vi "iteration.vi"(0 "GUI refnum cluster":T30, 1 "all settings":T1={"Variable Settings"={"Measurements per Iteration"=0, "Local Data Path"=path "", "Experiment description suffix for filename (no spaces please)"="", "Network Data Path"=path "", "Copy data to network"=FALSE, "Measurement Timeout (ms)"=0, "Independent Variables"=[], "Dependent Variables"=[], "Run Test Mode"=FALSE}, "HSDIO Settings"={"Enable HSDIO Pulses"=FALSE, "Resource Name"="", "Clock Rate"=0.0, "units/sec (ms=1000)"=0.0, "Array of Script Triggers"=[], "Channels Control"=[], "Pulse Generation Script"="", "Directory to look for waveform files"=path "", "Start Trigger"={"Wait for start trigger?"=FALSE, "source (PFI 0)"="", "edge (rising)"=0}, "Hardware alignment quantum\n(in samples)"=0, "Use file script"=FALSE, "Base path for script"=path "", "filename for script"=""}, "DAQmx Pulse Settings"={"Enable DAQmx Pulses"=FALSE, "DAQmx Physical Channels"="", "Clock Rate"=0.0, "units/sec (ms=1000)"=0.0, "Start Trigger"={"Wait for start trigger?"=FALSE, "source"="", "edge"=0}, "Timing Sequence Control"=[]}, "DDS Settings"={"Enable DDS"=FALSE, "Array of DDS Boxes"=[]}, "Camera settings"={"Analog Gain (0-5)"=0, "Frame Grabber acquisition region\n(left, top, right, bottom)"=[], "Exposure Time"=0.0, "EM Gain (0-255)"=0, "Trigger Polarity"="", "External Trigger Mode"="", "Scan Speed"="", "External Trigger Source"="", "Scan Mode"="", "Super Pixel Binning\n(if enabled in Scan Mode)"="", "Camera Sub-array acquisition region\n(if enabled in scan mode)"={"Left"=0, "Top"=0, "Width"=0, "Height"=0}, "Use camera?"=FALSE, "# image buffers"=0, "Regions of Interest (Left, Top, Right, Bottom)"=[], "Background Regions (Left, Top, Right, Bottom)"=[], "shots per measurement"=0, "Photoelectron Scaling"=0.0, "Force images to U16"=FALSE}, "Counter Settings"={"Enable Counters"=FALSE, "Array of Counter Settings"=[]}, "Filter Cluster"={"Counter Filter thresholds"=[], "Data Filters\nROI Minimum Thresholds"=[]}, "Analog Output Parameters"={"Enable Analog Out?"=TRUE, "Physical Channel"="PXI1Slot2/ao0:2", "Minimum Value"=-10.0, "Maximum Value"=10.0, "Samples per second"="", "Total AO Time (seconds)"="p", "Analog Output Equations for each Channel"=[], "Start Trigger"={"Wait for start trigger?"=FALSE, "source"="/Dev1/PFI0", "edge"=10280}}, "Notes"="", "HP83623A Generator Settings Array"=[], "Iteration Graph Settings"={"Plot Regions"="", "Plot Shots"=""}, "PI Piezo Settings"={"Enable"=FALSE, "Array of Piezo Controllers"=[]}, "Andor settings"={"Andor Path"=path "", "Copy any Andor files"=FALSE, "Wait time before copying Andor files (ms)"=0}, "Measurement Chart Settings"={"Which regions to plot (comma separated)"="", "Which shot to plot"=0}, "HP8662A Synthesized Signal Generator Array"=[], "HP83712B Synthesized CW Generator Array"=[], "TTL input"={"Enable"=FALSE, "lines"=""}} {"Variable Settings"."Independent Variables"."# steps" min=1 step=1; "Variable Settings"."Measurements per Iteration" min=1 step=1; "HSDIO Settings"."Hardware alignment quantum\n(in samples)" min=1 step=1; "HSDIO Settings"."Array of Script Triggers"."level" items=["High Level"=34, "Low Level"=35]; "HSDIO Settings"."Array of Script Triggers"."edge" items=["Rising Edge"=12, "Falling Edge"=13]; "HSDIO Settings"."Start Trigger"."edge (rising)" items=["Rising Edge"=12, "Falling Edge"=13]; "HSDIO Settings"."Clock Rate" min=0.0 max=200000000.0 format="%.2p"; "DAQmx Pulse Settings"."Start Trigger"."edge" items=["Rising"=10280, "Falling"=10171]; "DAQmx Pulse Settings"."Clock Rate" min=0.0 max=200000000.0 format="%.2p"; "Camera settings"."shots per measurement" min=0 step=1; "Camera settings"."Background Regions (Left, Top, Right, Bottom)" min=0 max=512 step=1; "Camera settings"."Regions of Interest (Left, Top, Right, Bottom)" min=0 max=512 step=1; "Camera settings"."# image buffers" min=0 step=1; "Camera settings"."Camera Sub-array acquisition region\n(if enabled in scan mode)"."Height" min=16 max=512 step=16; "Camera settings"."Camera Sub-array acquisition region\n(if enabled in scan mode)"."Width" min=16 max=512 step=16; "Camera settings"."Camera Sub-array acquisition region\n(if enabled in scan mode)"."Top" max=496 step=16; "Camera settings"."Camera Sub-array acquisition region\n(if enabled in scan mode)"."Left" max=496 step=16; "Camera settings"."Frame Grabber acquisition region\n(left, top, right, bottom)" min=0 max=512 step=1; "Camera settings"."Analog Gain (0-5)" max=5 step=1; "Counter Settings"."Array of Counter Settings"."Binwidth (ms)" format="%0.2f"; "Analog Output Parameters"."Start Trigger"."edge" items=["Rising"=10280, "Falling"=10171]; "Analog Output Parameters"."Maximum Value" format="%0.2f"; "Analog Output Parameters"."Minimum Value" format="%0.2f"}, 2 "Variable Settings Refnum":refnum<vi>, 7 "error in (no error)":errorcluster, 8 "Image Display Refnum Array":refnum<vi>[](array[refnum]), 12 "Camera Temperature Refnum":refnum<vi>, 14 "HSDIO Status Refnum":refnum<vi>, 16 "# intervals (mutli-shot)":i32=128, 17 "Notes Refnum":refnum<vi>, 22 "Hamamatsu_C9100-13.lvclass":refnum<class "Hamamatsu_C9100-13.lvclass">, 26 "Variable Status Refnum":refnum<vi>) -> (20 "Array of ROI sums":dbl[][][][](array[numeric])=[[[[-878.86977886979]]]], 21 "Image Array for whole experiment":T35[][][](array[plugin-control]) caption="(Cycles, Iterations, Measurements, Shots, scaling above)", 23 "Histogram of ROI Sum over All Images for last ROI":T33, 24 "Average of All Images from experiment":T35(plugin-control) caption="Average of All Images (dynamically scaled)", 25 "Camera out":refnum<class "Hamamatsu_C9100-13.lvclass">, 27 "error out":errorcluster)   [LabVIEW 2012]
doc: "I Description:\nThis example uses a script to manage the generation of a dynamic pattern at a specified clock rate.\n\nII Instructions for Running:\n1. Enter the digital channels on the hardware device to generate digital pattern in the Channel List control.\n2. Specify the clock rate for the generation in the Clock Rate control.\n3. Click the Stop button when you want to stop the generation\n\nIII Block Diagram Steps:\n1. Initialize for a generation session.\n2. Assign specified channels in Channel List for dynamic operation.\n3. Configure the Sample clock to use the onboard clock, and configure the clock rate.\n4. Set the generation mode to Scripted.\n5. Query the Data Width property to determine which Write function to use.\nNote: Different devices have different default values for the Data Width property. If you know the Data Width of your device, you may omit the property node and case structure.\n6. Write digital patterns to the onboard memory of the digital device.\n7. Write the script to the onboard memory.\n8. Initiate dynamic pattern generation.\n9. Wait until the Stop button is clicked or an error occurs, and exit the While loop. \n The niHSDIO Is Done VI is used in the while loop to check only for errors.\n10. Abort generation and close the session.\n\nIV I/O Connections Overview:\nMake connections from output terminals to match the channels specified by Channel List. In this example, the digital pattern is generated from the first 16 digital channels of the device."
uses:
  ExperimentVariables/ExperimentVariables.lvclass
  DAQmx_pulse_out/DAQmx_pulse_out.lvclass
  HSDIO/HSDIO.lvclass
  Analog_output/Analog_Output.lvclass
  Camera/Hamamatsu_C9100-13/Hamamatsu_C9100-13.lvclass
  Counter/Counter.lvclass
  GPIB/GPIB.lvclass
  Analog_output/AO_settings.ctl
  Camera/Hamamatsu_C9100-13/camera_setup.ctl
  DDS drivers v3/DDS RAM mode.ctl
  <vilib>/ni845x/ni845x.llb/ni845xControl.ctl
  <instrlib>/niHSDIO/niHSDIO.llb/niHSDIO_ctl Trigger Script - trigID Values (Ring).ctl
  <instrlib>/niHSDIO/niHSDIO.llb/niHSDIO_ctl Trigger DigEdge - Edge Values (Ring).ctl
  <instrlib>/niHSDIO/niHSDIO.llb/niHSDIO_ctl Trigger Source Values (Ring).ctl
  ExperimentVariables/Variable_Settings.ctl
  Counter/Counter_Settings_Control.ctl
  HSDIO/HSDIO_settings.ctl
  DAQmx_pulse_out/settings.ctl
  <instrlib>/niHSDIO/niHSDIO.llb/niHSDIO_ctl Trigger DigLvl - Level Values (Ring).ctl
  histogram.ctl
  gui_refnum.ctl
  Counter/counter_graph_refnums.ctl
  filters/filters.ctl
  gui_execution_controls.ctl
  DDS drivers v3/Array_of_DDS_Boxes.ctl
  DDS drivers v3/DDS_box_device_reference.ctl
  DDS drivers v3/DDS_box_cluster.ctl
  DDS/DDS_Settings_Cluster.ctl
  config_file_io/all_settings.ctl
  ExperimentVariables/Variable_Status.ctl
  GPIB/HP83623A_RF_Generator/HP83623A_settings.ctl
  GPIB/HP83623A_RF_Generator/HP83623A_RF_Generator.lvclass
  PI_piezo/settings.ctl
  PI_piezo/status.ctl
  Camera/Andor/Andor_settings.ctl
  gui/measurement_graph.ctl
  GPIB/RF_Generator_settings.ctl
  GPIB/RF_Generator_settings_array.ctl
  DDS drivers v3/DDS_profile.ctl
  DDS drivers v3/DDS_channel.ctl
  DDS/DDS.lvclass
  DDS drivers v3/array_of_DDS_profiles.ctl
  DDS drivers v3/array_of_DDS_channels.ctl
  ExperimentVariables/current_variables_table.ctl
  TTL_input/TTL_input_settings.ctl
  TTL_input/TTL_input.lvclass
panel:
  out "Counter out":refnum<class "Counter.lvclass">
  out "HSDIO":refnum<class "HSDIO.lvclass">
  out "Run Test Mode":bool
  in  "Tab Control":T34(tab)=enum."Filters"
  # "Parameters will be evaluated once at the beginning of the experiment from top to bottom, \nso any parameter may depend on all those above it.\nVariables will be evaluated each iteration.\nParameters and Variables may be used in various other experiment settings, as noted.\nSee LabView Help -> Formula Node and Expression Node Functions for a list of available functions."
  # "Parameters will be evaluated once at the beginning of the experiment from top to bottom, \nso any parameter may depend on all those above it.\nVariables will be evaluated each iteration.\nParameters and Variables may be used in various other experiment settings, as noted.\nSee LabView Help -> Formula Node and Expression Node Functions for a list of available functions."
  # "Regions of Interest -->"
  # "Shots\n   |\n  V"
  # "Counters -->"
  # "Counter\n    bins\n       |\n      V"
  # "You may use formulas here.  If 't' is not specified in the variable or parameter tables, it will be used here as time in seconds.\nIn addition to the usual functions (sin(), cos(), etc.) you may also use spike(), square() and step(), \nNote, analog output will continue until Total AO Time runs out, or Measurement Timeout is reached, \neven if HSDIO pulses or DAQmx pulses have finished."
  # "Notes will be auto-evaluated and will be saved with comments in each experiment directory."
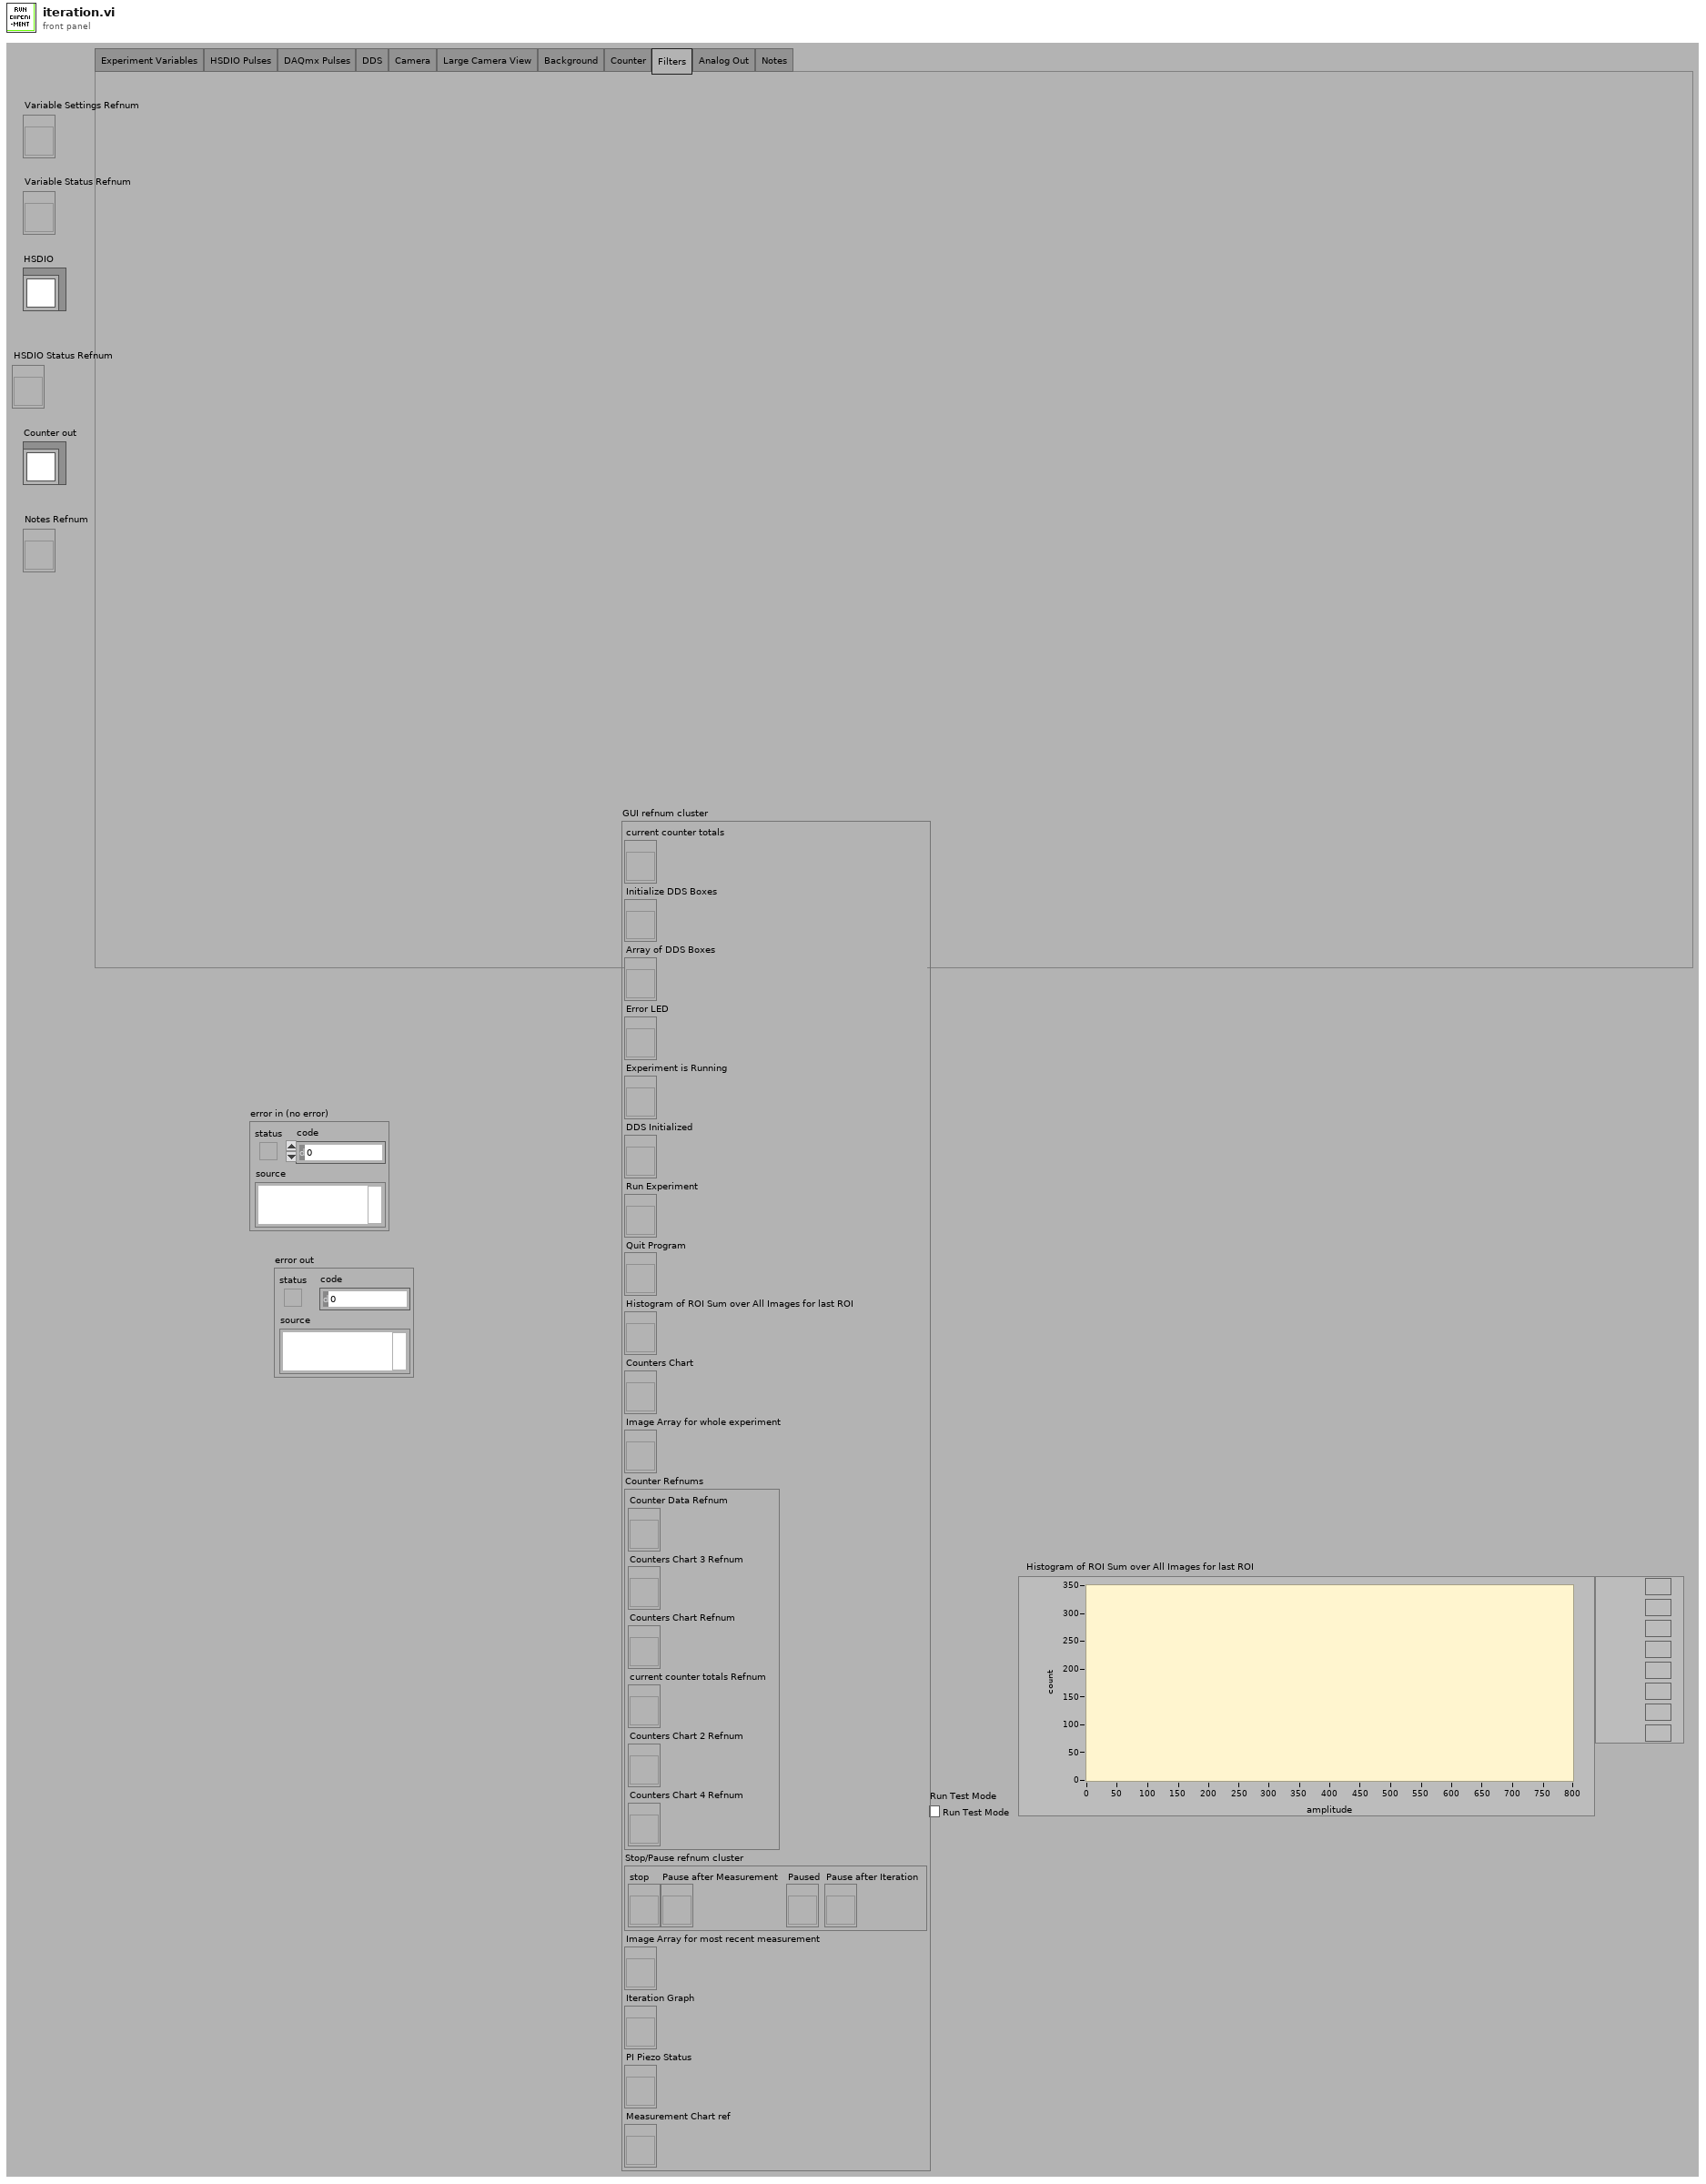
[diagram p1: front panel]
types:
  T1 = typedef "all_settings.ctl" = cluster{"Variable Settings":T2, "HSDIO Settings":T3, "DAQmx Pulse Settings":T8, "DDS Settings":T9, "Camera settings":T19, "Counter Settings":T20, "Filter Cluster":T21, "Analog Output Parameters":T22, "Notes":string, "HP83623A Generator Settings Array":T23, "Iteration Graph Settings":cluster{"Plot Regions":string, "Plot Shots":string}, "PI Piezo Settings":T24, "Andor settings":T25, "Measurement Chart Settings":T26, "HP8662A Synthesized Signal Generator Array":T27, "HP83712B Synthesized CW Generator Array":T27, "TTL input":T29}
  T2 = typedef "ExperimentVariables.lvclass/Variable_Settings.ctl" = cluster{"Measurements per Iteration":i32, "Local Data Path":path, "Experiment description suffix for filename (no spaces please)":string, "Network Data Path":path, "Copy data to network":bool, "Measurement Timeout (ms)":u32, "Independent Variables":cluster{"Description":string, "Name (a,a0...a9)":string, "min":dbl, "max":dbl, "# steps":u32}[], "Dependent Variables":cluster{"Description":string, "Name (a,a0...a9)":string, "Equation":string, "Result":dbl}[], "Run Test Mode":bool}
  T3 = typedef "HSDIO.lvclass/HSDIO_settings.ctl" = cluster{"Enable HSDIO Pulses":bool, "Resource Name":refnum<k15>, "Clock Rate":dbl, "units/sec (ms=1000)":dbl, "Array of Script Triggers":cluster{"trigger id (script trigger 0)":T4, "source (PFI 0)":T5, "Trigger Type":enum32{"Edge", "Level"}, "edge":T6, "level":T7}[], "Channels Control":string[][], "Pulse Generation Script":string, "Directory to look for waveform files":path, "Start Trigger":cluster{"Wait for start trigger?":bool, "source (PFI 0)":T5, "edge (rising)":T6}, "Hardware alignment quantum\n(in samples)":u16, "Use file script":bool, "Base path for script":path, "filename for script":string}
  T4 = typedef "niHSDIO_ctl Trigger Script - trigID Values (Ring).ctl" = string
  T5 = typedef "niHSDIO_ctl Trigger Source Values (Ring).ctl" = string
  T6 = typedef "niHSDIO_ctl Trigger DigEdge - Edge Values (Ring).ctl" = i32
  T7 = typedef "niHSDIO_ctl Trigger DigLvl - Level Values (Ring).ctl" = i32
  T8 = typedef "DAQmx_pulse_out.lvclass/settings.ctl" = cluster{"Enable DAQmx Pulses":bool, "DAQmx Physical Channels":tag, "Clock Rate":dbl, "units/sec (ms=1000)":dbl, "Start Trigger":cluster{"Wait for start trigger?":bool, "source":tag, "edge":i32}, "Timing Sequence Control":string[][]}
  T9 = typedef "DDS_Settings_Cluster.ctl" = cluster{"Enable DDS":bool, "Array of DDS Boxes":T10}
  T10 = typedef "Array_of_DDS_Boxes.ctl" = T11[]
  T11 = typedef "DDS_box_cluster.ctl" = cluster{"DDS box device reference":T12, "Array of DDS Channels (4)":T14, "Enable":bool, "Description":string}
  T12 = typedef "DDS_box_device_reference.ctl" = cluster{"NI USB-8451 device reference":T13, "DIO port":u8, "Serial Clock Rate [kHz]":u16}
  T13 = typedef "ni845xControl.ctl" = refnum<k21>
  T14 = typedef "DDS.lvclass/array_of_DDS_channels.ctl" = T15[]
  T15 = typedef "DDS.lvclass/DDS_channel.ctl" = cluster{"Power":bool, "Channel Parameters":cluster{"Ref Clock Rate [kHz]":dbl, "Full Scale Output\nPower [dBm]":dbl}, "RAM Enable":bool, "RAM Dest Type":u8, "RAM Default":cluster{"Frequency [MHz]":string, "Amplitude [dBm]":string, "Phase Offset [rad]":string}, "Array of DDS Profiles (8)":T16, "Description":string}
  T16 = typedef "DDS.lvclass/array_of_DDS_profiles.ctl" = T17[]
  T17 = typedef "DDS_profile.ctl" = cluster{"Single Tone":cluster{"Frequency [MHz]":string, "Amplitude [dBm]":string, "Phase Offset [rad]":string}, "RAM Mode ":T18, "Zero-crossing":bool, "No Dwell High":bool, "Function/Static":bool, "RAM Function Settings":string[], "RAM Static Array":dbl[], "Description":string}
  T18 = typedef "DDS RAM mode.ctl" = enum16{"Direct Switch", "Ramp Up", "Bidirectional Ramp", "Continuous Bidirectional Ramp", "Continuous Recirculate", "Direct Switch 2", "Direct Switch 3", "Direct Switch 4"}
  T19 = typedef "Hamamatsu_C9100-13.lvclass/camera_setup.ctl" = cluster{"Analog Gain (0-5)":u8, "Frame Grabber acquisition region\n(left, top, right, bottom)":i32[], "Exposure Time":dbl, "EM Gain (0-255)":u8, "Trigger Polarity":string, "External Trigger Mode":string, "Scan Speed":string, "External Trigger Source":string, "Scan Mode":string, "Super Pixel Binning\n(if enabled in Scan Mode)":string, "Camera Sub-array acquisition region\n(if enabled in scan mode)":cluster{"Left":u16, "Top":u16, "Width":u16, "Height":u16}, "Use camera?":bool, "# image buffers":i32, "Regions of Interest (Left, Top, Right, Bottom)":i32[][], "Background Regions (Left, Top, Right, Bottom)":i32[][], "shots per measurement":i32, "Photoelectron Scaling":dbl, "Force images to U16":bool}
  T20 = typedef "Counter.lvclass/Counter_Settings_Control.ctl" = cluster{"Enable Counters":bool, "Array of Counter Settings":cluster{"Counter Channel":tag, "Time-Bin Clock Channel":tag, "Binwidth (ms)":dbl}[]}
  T21 = typedef "filters.ctl" = cluster{"Counter Filter thresholds":u32[][], "Data Filters\nROI Minimum Thresholds":u64[][]}
  T22 = typedef "Analog_Output.lvclass/AO_settings.ctl" = cluster{"Enable Analog Out?":bool, "Physical Channel":tag, "Minimum Value":dbl, "Maximum Value":dbl, "Samples per second":string, "Total AO Time (seconds)":string, "Analog Output Equations for each Channel":string[], "Start Trigger":cluster{"Wait for start trigger?":bool, "source":tag, "edge":i32}}
  T23 = typedef "HP83623A_RF_Generator.lvclass/HP83623A_settings.ctl" = cluster{"Frequency (Hz)":string, "Power (dBm)":string, "Enabled":bool, "initialized":bool, "RF Output On/Off":bool, "External Trigger?":bool, "VISA Session":refnum<visa-resource-name>, "Generator Name":string}[]
  T24 = typedef "settings.ctl" = cluster{"Enable":bool, "Array of Piezo Controllers":cluster{"Enable":bool, "Serial No.":string, "Array of Piezo Channels":cluster{"Servo":bool, "Set Position":string}[]}[]}
  T25 = typedef "Andor_settings.ctl" = cluster{"Andor Path":path, "Copy any Andor files":bool, "Wait time before copying Andor files (ms)":u16}
  T26 = typedef "measurement_graph.ctl" = cluster{"Which regions to plot (comma separated)":string, "Which shot to plot":u8}
  T27 = typedef "GPIB.lvclass/RF_Generator_settings_array.ctl" = T28[]
  T28 = typedef "GPIB.lvclass/RF_Generator_settings.ctl" = cluster{"Enable":bool, "Description":string, "GPIB channel #":u8, "Frequency (MHz)":string, "Power (dBm)":string}
  T29 = typedef "TTL_input.lvclass/TTL_input_settings.ctl" = cluster{"Enable":bool, "lines":tag}
  T30 = typedef "gui_refnum.ctl" = cluster{"current counter totals":refnum<vi>, "Initialize DDS Boxes":refnum<vi>, "Array of DDS Boxes":refnum<vi>, "Error LED":refnum<vi>, "Experiment is Running":refnum<vi>, "DDS Initialized":refnum<vi>, "Run Experiment":refnum<vi>, "Quit Program":refnum<vi>, "Histogram of ROI Sum over All Images for last ROI":refnum<vi>, "Counters Chart":refnum<vi>, "Image Array for whole experiment":refnum<vi>, "Counter Refnums":T31, "Stop/Pause refnum cluster":T32, "Image Array for most recent measurement":refnum<vi>, "Iteration Graph":refnum<vi>, "PI Piezo Status":refnum<vi>, "Measurement Chart ref":refnum<vi>}
  T31 = typedef "counter_graph_refnums.ctl" = cluster{"Counter Data Refnum":refnum<vi>, "Counters Chart 3 Refnum":refnum<vi>, "Counters Chart Refnum":refnum<vi>, "current counter totals Refnum":refnum<vi>, "Counters Chart 2 Refnum":refnum<vi>, "Counters Chart 4 Refnum":refnum<vi>}
  T32 = typedef "gui_execution_controls.ctl" = cluster{"stop":refnum<vi>, "Pause after Measurement":refnum<vi>, "Paused":refnum<vi>, "Pause after Iteration":refnum<vi>}
  T33 = typedef "histogram.ctl" = cluster{"X Values":dbl[], "Histogram: h(x)":i32[]}[]
  T34 = enum32{"Experiment Variables", "HSDIO Pulses", "DAQmx Pulses", "DDS", "Camera", "Large Camera View", "Background", "Counter", "Filters", "Analog Out", "Notes"}
  T35 = typedef "IMAQ Image.ctl" = refnum<image>
  T36 = enum16{"reset", "experiment start", "experiment end", "quit"}
  T37 = cluster{"Plot Regions":string, "Plot Shots":string}
  T38 = cluster{"Global Rectangle":i32[], "Contours":cluster{"Contour Type":u32, "ROI Type":u32, "Points":i32[]}[]}
  T39 = cluster{"X Values":dbl[], "Histogram: h(x)":i32[]}[]
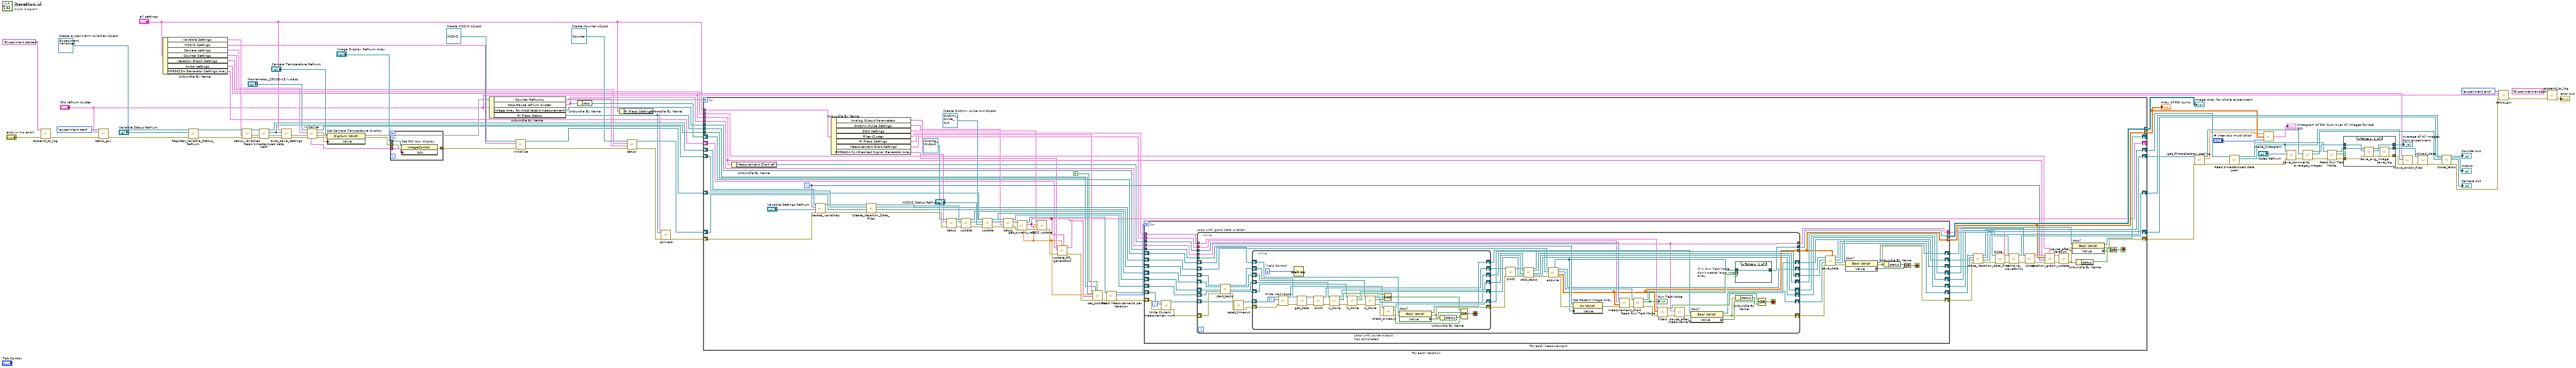
[diagram p0: block diagram]
diagram:
  w49 = refnum<class "Counter.lvclass"> refnum  # Create Counter object
  w77 = refnum<class "HSDIO.lvclass"> refnum  # Create HSDIO object
  w53 = refnum<class "ExperimentVariables.lvclass"> refnum  # Create experiment variables object
  n1 = call "append_to_log.vi"("error in"="error in (no error)", "string"="Experiment started") -> ("error out"=w58:errorcluster)  [unwired: 9 in]
  n2 = call "setup_gui.vi"("Enum"=T36."experiment start", "GUI refnum cluster"="GUI refnum cluster", "error in (no error)"=w58) -> ("error out"=w51:errorcluster)  [unwired: 12 in]
  n3 = Unbundle By Name("all settings") -> ("Variable Settings"=w18:T2, "HSDIO Settings"=w17:T3, "Camera settings"=w16:T19, "Counter Settings"=w15:T20, "Iteration Graph Settings"=w12:T37, "Andor settings"=w3:T25, "HP83623A Generator Settings Array"=w1:T23)
  n4 = call-dynamic "Register_Variable_Status_Refnum.vi"("error in (no error)"=w51, "Variable Status Refnum"="Variable Status Refnum", "ExperimentVariables in"=w53) -> ("error out"=w50:errorcluster, "ExperimentVariables out"=w52:refnum<class "ExperimentVariables.lvclass">)  [unwired: 7 in]
  n5 = call "setup_variables.vi"("error in (no error)"=w50, "Variable Settings"=w18, 11:w52) -> ("error out"=w39:errorcluster, 1:w79, "ExperimentVariables out"=w41:refnum<class "ExperimentVariables.lvclass">)  [unwired: 6 in]
  n6 = call-dynamic "Read timestamped data path.vi"("error in (no error)"=w39, "ExperimentVariables in"=w41) -> ("error out"=w19:errorcluster, "Specific Data Files Path"=w6:path, "ExperimentVariables out"=w40:refnum<class "ExperimentVariables.lvclass">)  [unwired: 7 in]
  n7 = call "auto_save_settings.vi"("error in"=w19, "base path"=w6, "all settings"="all settings") -> ("error out"=w14:errorcluster)  [unwired: 8 in]
  n8 = call-dynamic "initialize.vi"("error in (no error)"=w14, "Camera Setup"=w16, "Hamamatsu_C9100-13 in"="Hamamatsu_C9100-13.lvclass") -> ("error out"=w63:errorcluster, "Camera Temperature"=w64:dbl, "Hamamatsu_C9100-13 out"=w70:refnum<class "Hamamatsu_C9100-13.lvclass">, "ROI"=w71:T38)  [unwired: 5 in]
  n9 = property on="Set Camera Temperature Display" class="DigNum (strict)"(reference="Camera Temperature Refnum", error in=w63, "Value"=w64) -> (error out=w62:errorcluster)  [unwired: 1 out]
  n10 = for {
    tunnel: "Image Display Refnum Array" -> [w87] mode=indexing
    tunnel: w71 -> [w86]
    tunnel: w62 -> [w85]
    tunnel: [w84] -> w72
    n11 = property on="Set ROI box display" class="ImageControl"(reference=w87, error in=w85, "ROI"=w86) -> (error out=w84:errorcluster)  [unwired: 1 out]
  }
  n12 = Unbundle By Name("GUI refnum cluster") -> ("Counter Refnums"=w22:T31, "Stop/Pause refnum cluster"=w21:T32, "Image Array for most recent measurement"=w20:refnum<vi>, "PI Piezo Status"=w7:refnum<vi>)
  n13 = call "Initialize.vi"("error in (no error)"=w72, "HSDIO Settings"=w17, 11:w77) -> ("error out"=w48:errorcluster, "HSDIO out"=w76:refnum<class "HSDIO.lvclass">)  [unwired: 7 in]
  n14 = Unbundle By Name(w21) -> ("stop"=w61:refnum<vi>)
  n15 = Unbundle By Name("all settings") -> ("PI Piezo Settings"=w9:T24)
  n16 = call "setup.vi"("error in (no error)"=w48, "Counter Refnums"=w22, "Counter Settings"=w15, 11:w49) -> ("error out"=w11:errorcluster, "Counter out"=w47:refnum<class "Counter.lvclass">)  [unwired: 6 in]
  n17 = call "connect.vi"("PI Piezo Settings"=w9, "PI Piezo Status"=w7, "error in"=w11) -> ("error out"=w8:errorcluster)  [unwired: 16 in]
  n18 = for "For each Iteration" {
    N: w79 -> [_]
    shift-right: [w140] -> w27
    shift-left: w8 -> [w166]
    tunnel: [w108] -> w68 mode=indexing
    shift-right: [w162] -> w78
    shift-left: w76 -> [w165]
    shift-right: [w121] -> w80
    shift-left: w47 -> [w131]
    shift-right: [w124] -> w44
    shift-left: w40 -> [w167]
    tunnel: [w136] -> w75 mode=indexing
    shift-right: [w109] -> w28
    shift-left: w70 -> [w130]
    shift-right: [w138] -> _
    shift-left: w61 -> [w137]
    tunnel: w21 -> [w120]
    tunnel: w20 -> [w119]
    tunnel: "all settings" -> [w116]
    tunnel: "GUI refnum cluster" -> [w97]
    tunnel: w12 -> [w104]
    tunnel: w7 -> [w102]
    tunnel: w6 -> [w98]
    shift-right: [w89] -> _
    shift-left: w1 -> [w90]
    i -> [w105]
    stop <- w169 stop-if-true
    w160 = refnum<class "DAQmx_pulse_out.lvclass"> refnum  # Create DAQmx pulse out object
    n19 = Unbundle By Name(w97) -> ("Measurement Chart ref"=w96:refnum<vi>)
    n20 = call-dynamic "iterate_variables.vi"("error in (no error)"=w166, "Variable Settings Refnum"="Variable Settings Refnum", "Current Iteration"=w105, "ExperimentVariables in"=w167) -> ("error out"=w133:errorcluster, "ExperimentVariables out"=w135:refnum<class "ExperimentVariables.lvclass">)  [unwired: 6 in]
    n21 = Unbundle By Name(w116) -> ("Analog Output Parameters"=w113:T22, "DAQmx Pulse Settings"=w114:T8, "DDS Settings"=w115:T9, "Filter Cluster"=w112:T21, "PI Piezo Settings"=w103:T24, "Measurement Chart Settings"=w88:T26, "HP8662A Synthesized Signal Generator Array"=w95:T27)
    n22 = call-dynamic "Create_Iteration_Data_Files.vi"("error in (no error)"=w133, "Counter (in)"=w131, "Hamamatsu_C9100-13 (in)"=w130, "ExperimentVariables in"=w135) -> ("error out"=w132:errorcluster, "Counter out"=w128:refnum<class "Counter.lvclass">, "Hamamatsu_C9100-13"=w129:refnum<class "Hamamatsu_C9100-13.lvclass">, "ExperimentVariables out"=w134:refnum<class "ExperimentVariables.lvclass">)  [unwired: 4 in]
    n23 = call "setup.vi"("error in (no error)"=w132, "Analog Output Parameters"=w113, 11:refnum<class "Analog_Output.lvclass"> refnum ("Analog_Output.lvclass")) -> ("error out"=w143:errorcluster, "Analog_Output out"=w144:refnum<class "Analog_Output.lvclass">)  [unwired: 7 in]
    n24 = call-dynamic "update.vi"("error in (no error)"=w143, "ExperimentVariables (in)"=w134, "Analog_Output in"=w144) -> ("error out"=w149:errorcluster, "ExperimentVariables"=w147:refnum<class "ExperimentVariables.lvclass">, "Analog_Output out"=w148:refnum<class "Analog_Output.lvclass">)  [unwired: 6 in]
    n25 = call-dynamic "update.vi"("error in (no error)"=w149, "HSDIO Status Refnum"="HSDIO Status Refnum", "ExperimentVariables (in)"=w147, "HSDIO in"=w165) -> ("error out"=w110:errorcluster, "ExperimentVariables"=w158:refnum<class "ExperimentVariables.lvclass">, "HSDIO out"=w164:refnum<class "HSDIO.lvclass">)  [unwired: 5 in]
    n26 = call "setup.vi"("error in (no error)"=w110, "DAQmx Pulse Settings"=w114, "ExperimentVariables (in)"=w158, 11:w160) -> ("error out"=w159:errorcluster, "ExperimentVariables"=w157:refnum<class "ExperimentVariables.lvclass">, "DAQmx_pulse_out out"=w156:refnum<class "DAQmx_pulse_out.lvclass">)  [unwired: 5 in]
    n27 = call-dynamic "get_current_vars.vi"("error in (no error)"=w159, "ExperimentVariables in"=w157) -> ("error out"=w161:errorcluster, "variables and parameter names"=w91:string[], "ExperimentVariables out"=w151:refnum<class "ExperimentVariables.lvclass">, "current variable and parameter values"=w92:dbl[])  [unwired: 4 in, 2 out]
    n28 = call "DDS update.vi"("error in (no error)"=w161, "Variable Names"=w91, "Variable Values"=w92, "DDS Settings"=w115) -> ("error out"=w94:errorcluster)  [unwired: 7 in]
    n29 = call "update_RF_generators.vi"("variables and parameter names"=w91, "current variable and parameter values"=w92, "error in"=w94, "HP8662A Synthesized Signal Generator Array"=w95, "HP83623A Generator Settings Array (in)"=w90) -> ("error out"=w93:errorcluster, "HP83623A Generator Settings Array"=w89:T23)  [unwired: 5 in]
    n30 = call "set_position.vi"("PI Piezo Settings"=w103, "PI Piezo Status"=w102, "current variable and parameter values"=w92, "variables and parameter names"=w91, "error in"=w93, "file path"=w98, "Save positions?"=TRUE) -> ("error out"=w101:errorcluster)  [unwired: 12 in]
    n31 = call-dynamic "Read Measurements per Iteration.vi"("error in (no error)"=w101, "ExperimentVariables in"=w151) -> ("error out"=w152:errorcluster, "Measurements per Iteration"=w153:i32, "ExperimentVariables out"=w150:refnum<class "ExperimentVariables.lvclass">)  [unwired: 7 in]
    n32 = for "For each Measurement" {
      N: w153 -> [_]
      shift-right: [w204] -> w163
      shift-left: w164 -> [w205]
      shift-right: [w191] -> w127
      shift-left: w152 -> [w197]
      tunnel: [w184] -> w136 mode=indexing
      tunnel: [w185] -> w108 mode=indexing
      shift-right: [w192] -> w146
      shift-left: w148 -> [w193]
      shift-right: [w180] -> w122
      shift-left: w128 -> [w200]
      shift-right: [w198] -> w155
      shift-left: w156 -> [w199]
      shift-right: [w177] -> w125
      shift-left: w150 -> [w196]
      shift-right: [w178] -> w123
      shift-left: w129 -> [w203]
      shift-right: [w188] -> w139
      shift-left: w137 -> [w187]
      tunnel: w120 -> [w176]
      tunnel: w119 -> [w175]
      tunnel: [w174] -> w117
      tunnel: w112 -> [w172]
      tunnel: w96 -> [w171]
      tunnel: w88 -> [w170]
      i -> [w194]
      stop <- w201 stop-if-true
      n33 = call-dynamic "Write Current measuremen num.vi"("error in (no error)"=w197, "Current measurement #"=w194, "ExperimentVariables in"=w196) -> ("error out"=w186:errorcluster, "ExperimentVariables out"=w195:refnum<class "ExperimentVariables.lvclass">)  [unwired: 7 in]
      n34 = while "Loop until good data is taken" {
        tunnel: [w220] -> w184
        tunnel: [w206] -> w185
        shift-right: [w253] -> w204
        shift-left: w205 -> [w255]
        shift-right: [w230] -> w182
        shift-left: w186 -> [w244]
        shift-right: [w238] -> w192
        shift-left: w193 -> [w237]
        shift-right: [w249] -> w181
        shift-left: w200 -> [w251]
        shift-right: [w245] -> w198
        shift-left: w199 -> [w248]
        shift-right: [w217] -> w183
        shift-left: w195 -> [w241]
        shift-right: [w219] -> w179
        shift-left: w203 -> [w235]
        shift-right: [w229] -> w189
        shift-left: w187 -> [w232]
        tunnel: w175 -> [w215]
        tunnel: w176 -> [w214]
        tunnel: [w214] -> w174
        tunnel: w172 -> [w212]
        tunnel: w171 -> [w211]
        tunnel: w170 -> [w207]
        stop <- w256 stop-if-true
        n35 = call "start_tasks.vi"("Counter (in)"=w251, "Analog_Output in"=w237, "HSDIO (in)"=w255, "DAQmx_pulse_out (in)"=w248, "error in"=w244) -> ("Counter out"=w250:refnum<class "Counter.lvclass">, "Analog_Output"=w236:refnum<class "Analog_Output.lvclass">, "HSDIO"=w252:refnum<class "HSDIO.lvclass">, "DAQmx_pulse_out"=w247:refnum<class "DAQmx_pulse_out.lvclass">, "error out"=w243:errorcluster)  [unwired: 10 in]
        n36 = call-dynamic "reset_timeout.vi"("error in (no error)"=w243, "ExperimentVariables in"=w241) -> ("error out"=w242:errorcluster, "ExperimentVariables out"=w240:refnum<class "ExperimentVariables.lvclass">)  [unwired: 8 in]
        n37 = while "Loop until pulse output has completed" {
          shift-right: [w272] -> w210
          shift-left: w242 -> [w266]
          shift-right: [w289] -> w254
          shift-left: w252 -> [w290]
          shift-right: [w262] -> w225
          shift-left: w250 -> [w265]
          shift-right: [w287] -> w246
          shift-left: w247 -> [w288]
          shift-right: [w279] -> w239
          shift-left: w236 -> [w280]
          shift-right: [w285] -> w233
          shift-left: w240 -> [w268]
          shift-right: [w270] -> w213
          shift-left: w232 -> [w274]
          i -> [w269]
          stop <- w291 stop-if-true
          w292 = u32 1  # Yield Control
          n38 = call-dynamic "Write wait loops.vi"("error in (no error)"=w266, "wait loops"=w269, "ExperimentVariables in"=w268) -> ("error out"=w264:errorcluster, "ExperimentVariables out"=w267:refnum<class "ExperimentVariables.lvclass">)  [unwired: 7 in]
          n39 = Wait (ms)(milliseconds to wait=w292) -> ()  [unwired: 1 out]
          n40 = call-dynamic "get_data.vi"("error in (no error)"=w264, "Counter in"=w265) -> ("error out"=w261:errorcluster, "Counter out"=w263:refnum<class "Counter.lvclass">)  [unwired: 7 in, 1 out]
          n41 = call-dynamic "plot1.vi"("error in (no error)"=w261, "Counter in"=w263) -> ("error out"=w260:errorcluster, "Counter out"=w262:refnum<class "Counter.lvclass">)  [unwired: 8 in]
          n42 = call-dynamic "is_done.vi"("error in (no error)"=w260, "HSDIO in"=w290) -> ("error out"=w286:errorcluster, "HSDIO is done?"=w278:bool, "HSDIO out"=w289:refnum<class "HSDIO.lvclass">)  [unwired: 7 in]
          n43 = call-dynamic "is_done.vi"("error in (no error)"=w286, "DAQmx_pulse_out in"=w288) -> ("error out"=w282:errorcluster, "task done?"=w277:bool, "DAQmx_pulse_out out"=w287:refnum<class "DAQmx_pulse_out.lvclass">)  [unwired: 7 in]
          n44 = call-dynamic "is_done.vi"("error in (no error)"=w282, "Analog_Output in"=w280) -> ("error out"=w281:errorcluster, "task done?"=w275:bool, "Analog_Output out"=w279:refnum<class "Analog_Output.lvclass">)  [unwired: 7 in]
          n45 = call-dynamic "check_timeout.vi"("error in (no error)"=w281, "ExperimentVariables in"=w267) -> ("error out"=w273:errorcluster, "timeout elapsed?"=w283:bool, "ExperimentVariables out"=w285:refnum<class "ExperimentVariables.lvclass">)  [unwired: 7 in]
          n46 = Compound Arithmetic op=AND(w278, w277, w275) -> (w276:bool)
          n47 = property on="stop?" class="Bool (strict)"(reference=w274, error in=w273) -> (reference out=w270:refnum<vi>, error out=w272:errorcluster, "Value"=w271:bool)
          n48 = Unbundle By Name(w272) -> ("status"=w284:bool)
          n49 = Compound Arithmetic op=OR(w276, w271, w283, w284) -> (w291:bool)
        }
        n50 = call-dynamic "plot2.vi"("error in (no error)"=w210, "Counter in"=w225) -> ("error out"=w223:errorcluster, "Counter out"=w224:refnum<class "Counter.lvclass">)  [unwired: 8 in]
        n51 = call "stop_tasks.vi"("Counter (in)"=w224, "Analog_Output (in)"=w239, "HSDIO (in)"=w254, "DAQmx_pulse_out (in)"=w246, "error in"=w223) -> ("Counter"=w249:refnum<class "Counter.lvclass">, "Analog_Output"=w238:refnum<class "Analog_Output.lvclass">, "HSDIO"=w253:refnum<class "HSDIO.lvclass">, "DAQmx_pulse"=w245:refnum<class "DAQmx_pulse_out.lvclass">, "error out"=w234:errorcluster)  [unwired: 10 in]
        n52 = call-dynamic "acquire.vi"("error in (no error)"=w234, "ExperimentVariables (in)"=w233, "Hamamatsu_C9100-13 in"=w235) -> ("error out"=w228:errorcluster, "Array of ROI sums"=w206:dbl[][], "ExperimentVariables"=w218:refnum<class "ExperimentVariables.lvclass">, "Hamamatsu_C9100-13 out"=w219:refnum<class "Hamamatsu_C9100-13.lvclass">, "Image Array"=w221:T35[])  [unwired: 4 in]
        n53 = property on="Set Recent Image Array" class="Arr (strict)"(reference=w215, error in=w228, "Value"=w221) -> (error out=w209:errorcluster)  [unwired: 1 out]
        n54 = call "measurement_chart.vi"("error in"=w209, "Array of ROI"=w206, "Measurement Chart Settings"=w207, "Measurement Chart"=w211) -> ("error out"=w208:errorcluster)  [unwired: 7 in]
        n55 = call-dynamic "Read Run Test Mode.vi"("error in (no error)"=w208, "ExperimentVariables in"=w218) -> ("error out"=w216:errorcluster, "Run Test Mode"=w222:bool, "ExperimentVariables out"=w217:refnum<class "ExperimentVariables.lvclass">)  [unwired: 7 in]
        "Run Test Mode" <- w222
        n56 = call "filters.vi"("error in"=w216, "Array of ROI sums"=w206, "Filter Cluster"=w212) -> ("error out"=w227:errorcluster, "All shots passed filters?"=w257:bool)  [unwired: 7 in]
        n57 = call "pause_after_measurement.vi"("error in (no error)"=w227, 10:w214) -> ("error out"=w226:errorcluster)  [unwired: 9 in]
        n58 = property on="stop?" class="Bool (strict)"(reference=w213, error in=w226) -> (reference out=w229:refnum<vi>, error out=w230:errorcluster, "Value"=w231:bool)
        n59 = case "If in Run Test Mode,\ndon't create large image array." shown="False" w222 {
          tunnel: w221 -> [w259 _]
          tunnel: [w259 _] -> w220
          frame False {
          }
          frame True {
          }
        }
        n60 = Unbundle By Name(w230) -> ("status"=w258:bool)
        n61 = Compound Arithmetic op=OR(w257, w231, w258) -> (w256:bool)
      }
      n62 = call "save_data.vi"("Array of ROI sums"=w185, "error in (no error)"=w182, "ExperimentVariables (in)"=w183, "Counter (in)"=w181, "Camera (in)"=w179) -> ("error out"=w173:errorcluster, "ExperimentVariables"=w177:refnum<class "ExperimentVariables.lvclass">, "Counter"=w180:refnum<class "Counter.lvclass">, "Camera"=w178:refnum<class "Hamamatsu_C9100-13.lvclass">)  [unwired: 3 in]
      n63 = property on="stop?" class="Bool (strict)"(reference=w189, error in=w173) -> (reference out=w188:refnum<vi>, error out=w191:errorcluster, "Value"=w190:bool)
      n64 = Unbundle By Name(w191) -> ("status"=w202:bool)
      n65 = Or(x=w202, y=w190) -> (x .or. y?=w201:bool)
    }
    n66 = call-dynamic "close_iteration_data_files.vi"("error in (no error)"=w127, "Hamamatsu_C9100-13 (in)"=w123, "Counter (in)"=w122, "ExperimentVariables in"=w125) -> ("error out"=w126:errorcluster, "Hamamatsu_C9100-13"=w109:refnum<class "Hamamatsu_C9100-13.lvclass">, "Counter out"=w121:refnum<class "Counter.lvclass">, "ExperimentVariables out"=w124:refnum<class "ExperimentVariables.lvclass">)  [unwired: 4 in]
    n67 = call-dynamic "close.vi"("error in (no error)"=w126, "DAQmx_pulse_out in"=w155) -> ("error out"=w154:errorcluster)  [unwired: 8 in, 1 out]
    n68 = call-dynamic "remove_waveforms.vi"("error in (no error)"=w154, "HSDIO in"=w163) -> ("error out"=w145:errorcluster, "HSDIO out"=w162:refnum<class "HSDIO.lvclass">)  [unwired: 8 in]
    n69 = call-dynamic "close.vi"("error in (no error)"=w145, "Analog_Output in"=w146) -> ("error out"=w107:errorcluster)  [unwired: 8 in, 1 out]
    n70 = call "iteration_graph_update.vi"("Iteration Graph Settings"=w104, "error in (no error)"=w107, "Iteration Number"=w105, "ROI Array In"=w108, "GUI refnum cluster"=w97) -> ("error out"=w106:errorcluster)  [unwired: 5 in, 1 out]
    n71 = call "pause_after_iteration.vi"("error in (no error)"=w106, 11:w117) -> ("error out"=w118:errorcluster)  [unwired: 9 in]
    n72 = property on="stop?" class="Bool (strict)"(reference=w139, error in=w118) -> (reference out=w138:refnum<vi>, error out=w140:errorcluster, "Value"=w141:bool)
    n73 = Unbundle By Name(w118) -> ("status"=w168:bool)
    n74 = Or(x=w168, y=w141) -> (x .or. y?=w169:bool)
  }
  "Image Array for whole experiment" <- w75
  "Array of ROI sums" <- w68
  n75 = call-dynamic "get_Photoelectron_scaling.vi"("error in (no error)"=w27, "Hamamatsu_C9100-13 in"=w28) -> ("error out"=w26:errorcluster, "Photoelectron Scaling"=w24:dbl, "Hamamatsu_C9100-13 out"=w25:refnum<class "Hamamatsu_C9100-13.lvclass">)  [unwired: 7 in]
  n76 = call-dynamic "Read timestamped data path.vi"("error in (no error)"=w26, "ExperimentVariables in"=w44) -> ("error out"=w42:errorcluster, "Specific Data Files Path"=w2:path, "ExperimentVariables out"=w31:refnum<class "ExperimentVariables.lvclass">)  [unwired: 7 in]
  n77 = call "make_histogram.vi"("# intervals (mutli-shot)"="# intervals (mutli-shot)", "Array of ROI sums"=w68, "Photoelectron Scaling"=w24) -> ("Histogram over all images, for each region"=→"Histogram of ROI Sum over All Images for last ROI":T39)
  n78 = call "save_comments.vi"("error in"=w42, "Str Refnum"="Notes Refnum", "base path"=w2) -> ("error out"=w32:errorcluster)  [unwired: 8 in]
  n79 = call "average_images.vi"("error in (no error)"=w32, "Hamamatsu_C9100-13 (in)"=w25) -> ("error out"=w34:errorcluster, "Hamamatsu_C9100-13 out"=w69:refnum<class "Hamamatsu_C9100-13.lvclass">, "Average of Images"=w36:T35)  [unwired: 7 in]
  n80 = call-dynamic "Read Run Test Mode.vi"("error in (no error)"=w34, "ExperimentVariables in"=w31) -> ("error out"=w37:errorcluster, "Run Test Mode"=w38:bool, "ExperimentVariables out"=w33:refnum<class "ExperimentVariables.lvclass">)  [unwired: 7 in]
  n81 = case shown="False" w38 {
    tunnel: w37 -> [w294 w302]
    tunnel: w36 -> [w298 w303]
    tunnel: [w297 w303] -> w35
    tunnel: [w299 w302] -> w5
    tunnel: w33 -> [w296 w301]
    tunnel: [w300 w301] -> w30
    frame False {
      n82 = call "save_avg_image.vi"("error in (no error)"=w294, "Image"=w298, "ExperimentVariables in"=w296) -> ("error out"=w293:errorcluster, "Image Out (duplicate)"=w297:T35, "ExperimentVariables out"=w295:refnum<class "ExperimentVariables.lvclass">)  [unwired: 6 in]
      n83 = call "save_log.vi"("error in"=w293, "ExperimentVariables in"=w295) -> ("error out"=w299:errorcluster, "ExperimentVariables out"=w300:refnum<class "ExperimentVariables.lvclass">)  [unwired: 8 in]
    }
    frame True {
    }
  }
  "Average of All Images from experiment" <- w35
  n84 = call "move_andor_files.vi"("error in"=w5, "Data Files Path"=w2, "Andor setup"=w3) -> ("error out"=w4:errorcluster)  [unwired: 8 in]
  n85 = call-dynamic "upload_data.vi"("error in (no error)"=w4, "ExperimentVariables in"=w30) -> ("error out"=w29:errorcluster)  [unwired: 8 in, 1 out]
  n86 = call "close_tasks.vi"("Counter (in)"=w80, "HSDIO (in)"=w78, "Camera (in)"=w69, "error in"=w29) -> ("Counter"=→"Counter out":refnum<class "Counter.lvclass">, "HSDIO"=→"HSDIO":refnum<class "HSDIO.lvclass">, "Camera"=→"Camera out":refnum<class "Hamamatsu_C9100-13.lvclass">, "error out"=w81:errorcluster)  [unwired: 11 in, 1 out]
  n87 = call "setup_gui.vi"("Enum"=T36."experiment end", "GUI refnum cluster"="GUI refnum cluster", "error in (no error)"=w81) -> ("error out"=w56:errorcluster)  [unwired: 12 in]
  n88 = call "append_to_log.vi"("error in"=w56, "string"="Experiment ended") -> ("error out"=→"error out":errorcluster)  [unwired: 9 in]
